vi "IPS Set Target Current Sweep Rate.vi"(4 "Error In":errorcluster, 6 "Target Current Sweep Rate (A/min)":dbl, 7 "VISA resource name":refnum<visa-resource-name>="COM3") -> (0 "Error Out":errorcluster, 2 "read buffer":string, 3 "VISA resource name 2":refnum<visa-resource-name>="GPIB1::25::INSTR")   [LabVIEW 2016, in "IPS-120.lvlib"]
uses:
  IPS-120.lvlib
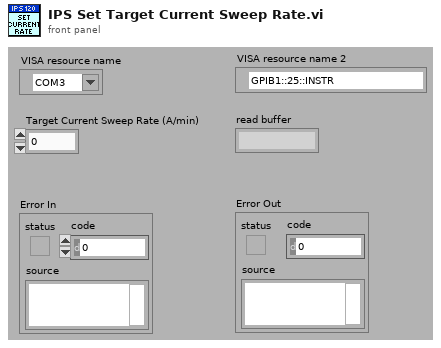
[diagram p1: front panel]
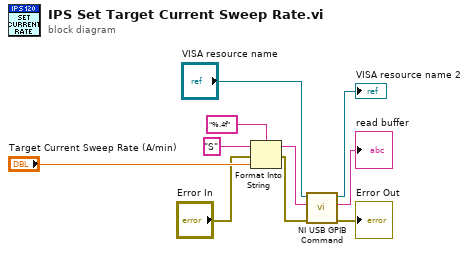
[diagram p0: block diagram]
diagram:
  n1 = Format Into String(format string="%.4f", initial string="S" ("string (\"\")"), error in="Error In", "Target Current Sweep Rate (A/min)") -> (resulting string=w6:string, error out=w1:errorcluster)
  n2 = call "NI USB GPIB Command.vi"("Error In"=w1, "write buffer"=w6, "VISA resource name"="VISA resource name") -> ("Error Out"=→"Error Out":errorcluster, "read buffer"=→"read buffer":string, "VISA resource name out"=→"VISA resource name 2":refnum<visa-resource-name>)  [unwired: 6 in]
